vi "Lire Operations.vi"(11 "Portfolio en entrée":refnum<class "Portfolio.lvclass">) -> (2 "Operations.lvclass":refnum<class "Operations.lvclass">, 3 "Portfolio en sortie":refnum<class "Portfolio.lvclass">)   [LabVIEW 2012, in "Portfolio.lvclass"]
uses:
  Portfolio.lvclass
  Operations/Operations.lvclass
  Portfolio.lvclass/Portfolio.ctl
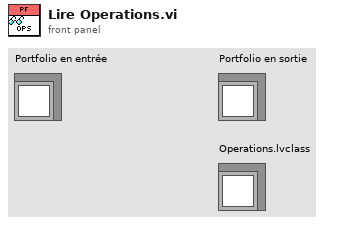
[diagram p1: front panel]
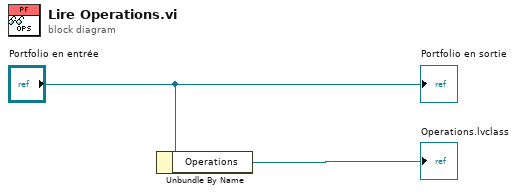
[diagram p0: block diagram]
diagram:
  n1 = Unbundle By Name("Portfolio en entrée") -> ("Operations"=→"Operations.lvclass":refnum<class "Operations.lvclass">)
  "Portfolio en sortie" <- "Portfolio en entrée"
